vi "Make a pre-header.vi"(2 "Row":T1={"Start"=0.0, "Start Caption"="Start [T]", "End"=0.0, "End Caption"="End [T]", "Sweep"=0.0, "Sweep caption"="Rate [mT/s]", "Constant"=0.0, "Constant caption"="Freq [GHz]", "Mod_F [kHz]"=0.0, "Mod_A [G]"=0.0, "Tau [ms]"=0.0, "Positioners [mm|°]"=[], "Tmp [K]"=50.0, "Wait [min]"=0.0, "Carousel"=-1, "Comment"="", "Auto-mod"=TRUE, "Execute"=FALSE} {"Carousel" items=["0", "1", "2", "3", "4", "5", "6"]; "Positioners [mm|°]" min=-1.0 max=330.0; "Tau [ms]" min=0.002 max=10000.0; "Wait [min]" min=0.0 max=3000.0; "Tmp [K]" min=0.0 max=350.0; "Mod_A [G]" min=0.0 max=100.0; "Mod_F [kHz]" min=0.1 max=150.0}, 3 "Add to heder comment":string) -> (0 "Pre-header string":string)   [LabVIEW 2022 SP3]
uses:
  Datatypes/script polymorh line.ctl
panel:
  out "error IO":errorcluster
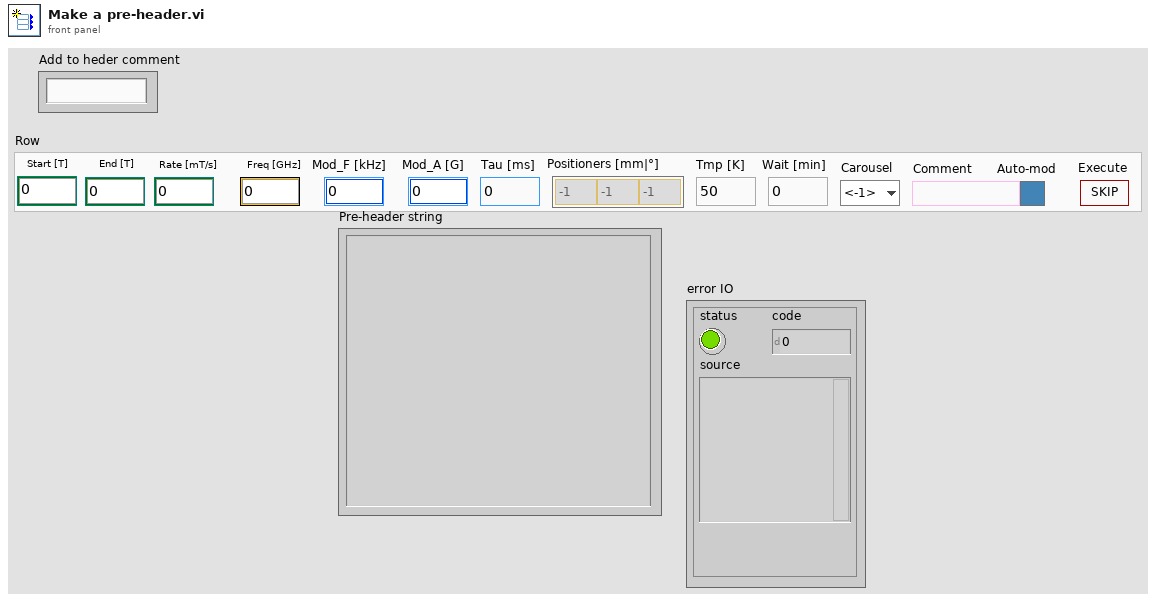
[diagram p1: front panel]
types:
  T1 = typedef "script polymorh line.ctl" = cluster{"Start":dbl, "Start Caption":string, "End":dbl, "End Caption":string, "Sweep":dbl, "Sweep caption":string, "Constant":dbl, "Constant caption":string, "Mod_F [kHz]":dbl, "Mod_A [G]":dbl, "Tau [ms]":dbl, "Positioners [mm|°]":dbl[], "Tmp [K]":dbl, "Wait [min]":dbl, "Carousel":i8, "Comment":string, "Auto-mod":bool, "Execute":bool}
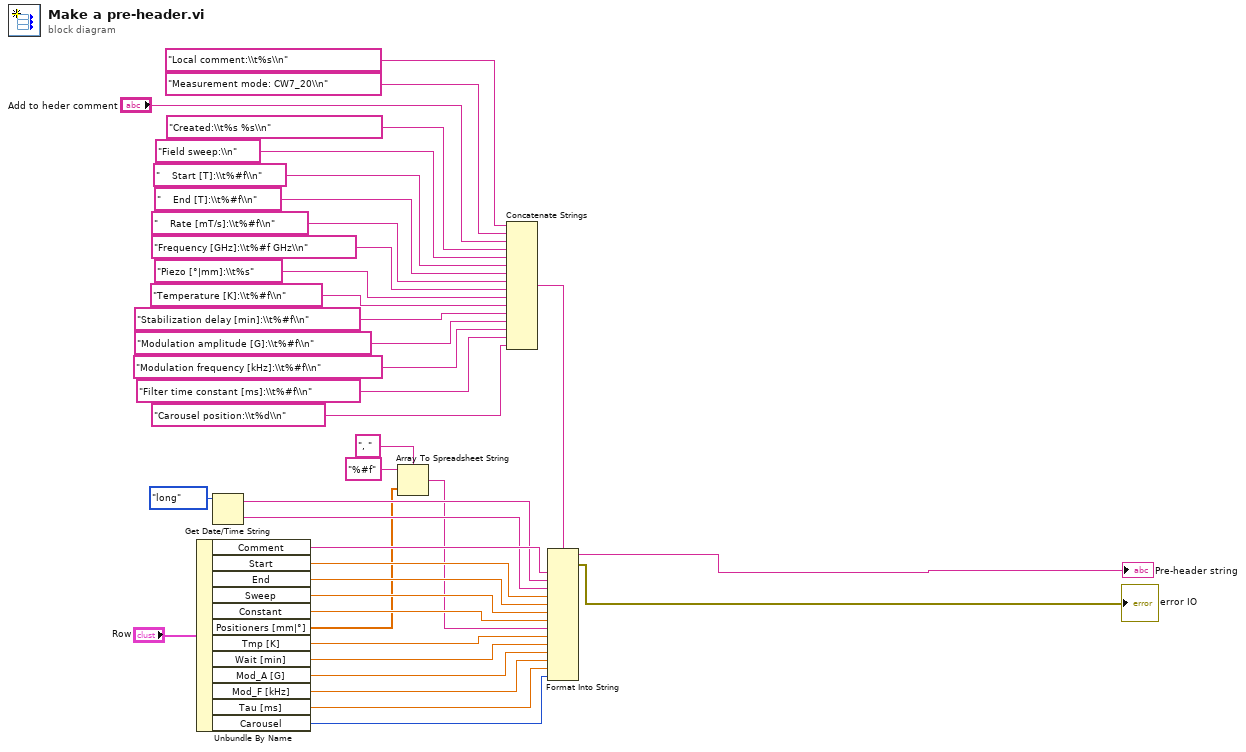
[diagram p0: block diagram]
diagram:
  n1 = Unbundle By Name("Row") -> ("Comment"=w10:string, "Start"=w17:dbl, "End"=w37:dbl, "Sweep"=w36:dbl, "Constant"=w35:dbl, "Positioners [mm|°]"=w2:dbl[], "Tmp [K]"=w34:dbl, "Wait [min]"=w21:dbl, "Mod_A [G]"=w20:dbl, "Mod_F [kHz]"=w19:dbl, "Tau [ms]"=w13:dbl, "Carousel"=w15:i8)
  n2 = Get Date/Time String(date format (0)=enum16{"short", "long", "abbreviated"}."long") -> (date string=w9:string, time string=w8:string)  [unwired: 2 in]
  n3 = Array To Spreadsheet String(delimiter (Tab)=", ", array=w2, 3:"%#f" ("format string")) -> (spreadsheet string=w1:string)
  n4 = Concatenate Strings("Local comment:\\t%s\\n", "Measurement mode: CW7_20\\n", "Add to heder comment", "Created:\\t%s %s\\n", "Field sweep:\\n", "    Start [T]:\\t%#f\\n", "    End [T]:\\t%#f\\n", "    Rate [mT/s]:\\t%#f\\n", "Frequency [GHz]:\\t%#f GHz\\n", "Piezo [°|mm]:\\t%s", "Temperature [K]:\\t%#f\\n", "Stabilization delay [min]:\\t%#f\\n" ("string"), "Modulation amplitude [G]:\\t%#f\\n" ("string"), "Modulation frequency [kHz]:\\t%#f\\n" ("string"), "Filter time constant [ms]:\\t%#f\\n" ("string"), "Carousel position:\\t%d\\n" ("string")) -> (w18:string)
  n5 = Format Into String(format string=w18, w10, w9, w8, w17, w37, w36, w35, w1, w34, w21, w20, w19, w13, w15) -> (resulting string=→"Pre-header string":string, error out=→"error IO":errorcluster)  [unwired: 2 in]
